vi "Start RUS Sweep.vi"(8 "error in (no error)":errorcluster, 11 "RUS Measurement in":refnum<class "RUS Measurement.lvclass">) -> (0 "error out":errorcluster, 3 "RUS Measurement out":refnum<class "RUS Measurement.lvclass">)   [LabVIEW 2015, in "RUS Measurement.lvclass"]
uses:
  RUS Measurement.lvclass
  RUS Parameters.ctl
  Hardware/Spectrum Analyzer Messages/Write Duration Msg/Write Duration Msg.lvclass
  Hardware/Spectrum Analyzer Messages/Write Frequencies Msg/Write Frequencies Msg.lvclass
  Hardware/Spectrum Analyzer Messages/Write Group Name Msg/Write Group Name Msg.lvclass
  Mag Lab Root/Mag Lab Root.lvclass/Mag Lab Root.ctl
  RUS Measurement.lvclass/RUS Measurement.ctl
  <vilib>/ActorFramework/Actor/Actor.lvclass/Actor.ctl
  Hardware/Spectrum Analyzer Messages/Write Duration Msg/Write Duration Msg.lvclass/Write Duration Msg.ctl
  Hardware/Spectrum Analyzer Messages/Write Frequencies Msg/Write Frequencies Msg.lvclass/Write Frequencies Msg.ctl
  Hardware/Spectrum Analyzer Messages/Write Group Name Msg/Write Group Name Msg.lvclass/Write Group Name Msg.ctl
  Mag Lab Measure Base Messages/Transmit Message Msg/Transmit Message Msg.lvclass/Transmit Message Msg.ctl
  <vilib>/ActorFramework/Message Enqueuer/Message Enqueuer.lvclass/Message Enqueuer.ctl
  Mag Lab Root Messages/Initialize Msg/Initialize Msg.lvclass/Initialize Msg.ctl
  Mag Lab Root/Read Name.vi
  Write Active.vi
  Write Sweep chunk.vi
  Read RUS Instrument.vi
  Mag Lab Root/Read Request time.vi
  <vilib>/ActorFramework/Message Enqueuer/Enqueue.vi
  <vilib>/ActorFramework/Message Priority Queue/Priority Enqueue.vi
  Mag Lab Properties/Mag Lab Parameters.lvclass
  Mag Lab Measure Base Messages/Transmit Message Msg/Transmit Message Msg.lvclass
  Mag Lab Root Messages/Initialize Msg/Initialize Msg.lvclass
  <vilib>/ActorFramework/Actor/Actor.lvclass
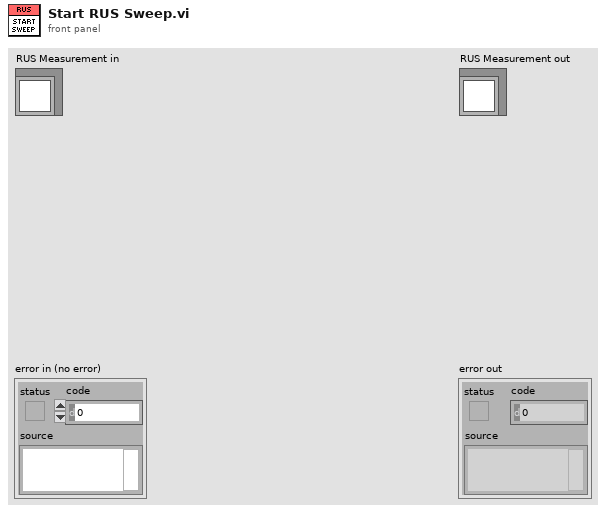
[diagram p1: front panel]
types:
  T1 = typedef "RUS Parameters.ctl" = cluster{"Start frequency":dbl, "End frequency":dbl, "Duration":dbl, "Averaging":dbl, "Find peaks":bool}
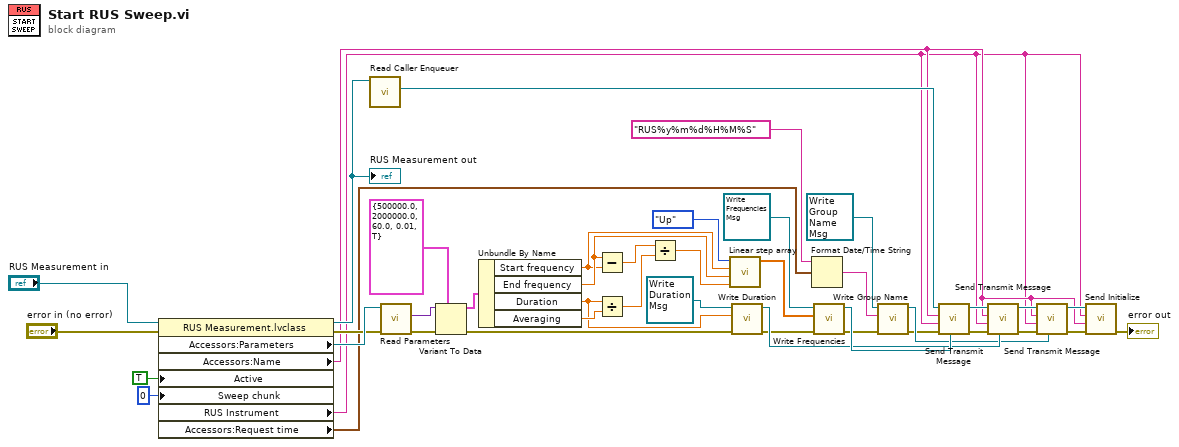
[diagram p0: block diagram]
diagram:
  n1 = property class="RUS Measurement.lvclass"(reference="RUS Measurement in", error in="error in (no error)", "Active"=TRUE, "Sweep chunk"=0) -> (reference out=w18:refnum<class "RUS Measurement.lvclass">, error out=w15:errorcluster, "Accessors:Parameters"=w16:refnum<class "Mag Lab Parameters.lvclass">, "Accessors:Name"=w5:string, "RUS Instrument"=w4:string, "Accessors:Request time"=w13:timestamp)
  "RUS Measurement out" <- w18
  n2 = call <vilib>:"Read Caller Enqueuer.vi"("Actor"=w18) -> ("Caller Enqueuer"=w21:refnum<class "Message Enqueuer.lvclass">)  [unwired: 10 in]
  n3 = call-dynamic "Read Parameters.vi"("error in (no error)"=w15, "Mag Lab Parameters in"=w16) -> ("error out"=w40:errorcluster, "Parameters"=w39:variant)  [unwired: 7 in, 1 out]
  n4 = Variant To Data(error in=w40, type=T1 {"Start frequency"=500000.0, "End frequency"=2000000.0, "Duration"=60.0, "Averaging"=0.01, "Find peaks"=TRUE} ("Parameters"), Variant=w39) -> (data=w37:T1, error out=w22:errorcluster)
  n5 = Unbundle By Name(w37) -> ("Start frequency"=w34:dbl, "End frequency"=w35:dbl, "Duration"=w27:dbl, "Averaging"=w36:dbl)
  n6 = Subtract(x=w35, y=w34) -> (x-y=w33:dbl)
  n7 = Divide(x=w27, y=w36) -> (x/y=w32:dbl)
  n8 = Divide(x=w33, y=w32) -> (x/y=w31:dbl)
  n9 = call "Linear step array.vi"("Step"=w31, "End"=w35, "Start"=w34, "Mode"=enum16{"Up", "Up-down"}."Up") -> ("Steps"=w29:dbl[])  [unwired: 7 in]
  n10 = call "Write Duration.vi"("error in (no error)"=w22, "Duration"=w27, "Write Duration Msg in"=refnum<class "Write Duration Msg.lvclass"> refnum ("Write Duration Msg.lvclass")) -> ("error out"=w23:errorcluster, "Write Duration Msg out"=w24:refnum<class "Write Duration Msg.lvclass">)  [unwired: 7 in]
  n11 = Format Date/Time String(time format string (%c)="RUS%y%m%d%H%M%S", seconds (now)=w13) -> (date/time string=w11:string)  [unwired: 1 in]
  n12 = call "Write Frequencies.vi"("error in (no error)"=w23, "Frequencies"=w29, "Write Frequencies Msg in"=refnum<class "Write Frequencies Msg.lvclass"> refnum ("Write Frequencies Msg.lvclass")) -> ("error out"=w10:errorcluster, "Write Frequencies Msg out"=w26:refnum<class "Write Frequencies Msg.lvclass">)  [unwired: 7 in]
  n13 = call "Write Group Name.vi"("error in (no error)"=w10, "Group Name"=w11, "Write Group Name Msg in"=refnum<class "Write Group Name Msg.lvclass"> refnum ("Write Group Name Msg.lvclass")) -> ("error out"=w2:errorcluster, "Write Group Name Msg out"=w3:refnum<class "Write Group Name Msg.lvclass">)  [unwired: 7 in]
  n14 = call "Send Transmit Message.vi"("Message"=w26, "error in (no error)"=w2, "Requestee"=w4, "Requestor"=w5, "Message Enqueuer"=w21) -> ("error out"=w25:errorcluster, "Message Enqueuer out"=w19:refnum<class "Message Enqueuer.lvclass">)  [unwired: 5 in]
  n15 = call "Send Transmit Message.vi"("Message"=w24, "error in (no error)"=w25, "Requestee"=w4, "Requestor"=w5, "Message Enqueuer"=w19) -> ("error out"=w9:errorcluster, "Message Enqueuer out"=w7:refnum<class "Message Enqueuer.lvclass">)  [unwired: 5 in]
  n16 = call "Send Transmit Message.vi"("Message"=w3, "error in (no error)"=w9, "Requestee"=w4, "Requestor"=w5, "Message Enqueuer"=w7) -> ("error out"=w8:errorcluster, "Message Enqueuer out"=w6:refnum<class "Message Enqueuer.lvclass">)  [unwired: 5 in]
  n17 = call "Send Initialize.vi"("error in (no error)"=w8, "Requestor"=w5, "Requestee"=w4, "Message Enqueuer"=w6) -> ("error out"=→"error out":errorcluster)  [unwired: 6 in, 1 out]
